vi "Array_filler.vi"() -> ()   [LabVIEW 2019]
panel:
  out "Indeks MAX":dbl[](array[numeric])
  out "Indeks MIN":dbl[](array[numeric])
  out "Rozmiar tablicy":dbl[](array[numeric])
  out "Suma":dbl
  out "Wartość MIN":dbl
  out "Wartość MAX":dbl
  in  "STOP":bool
  in  "Indeks kolumny":dbl
  in  "Indeks wiersza":dbl
  in  "Wypełnienie tablicy wstawianej":dbl
  out "Tablica wyjściowa":dbl[][](array[numeric])
  out "Tablica wstawiana":dbl[][](array[numeric])
  in  "Wprowadzanie danych":dbl[][](array[numeric])
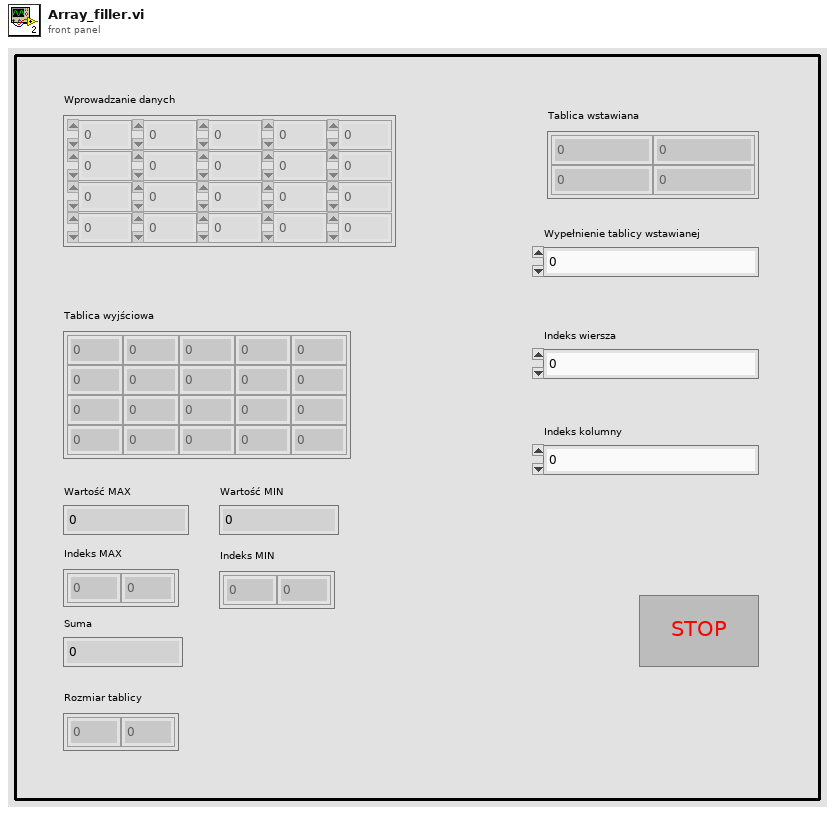
[diagram p1: front panel]
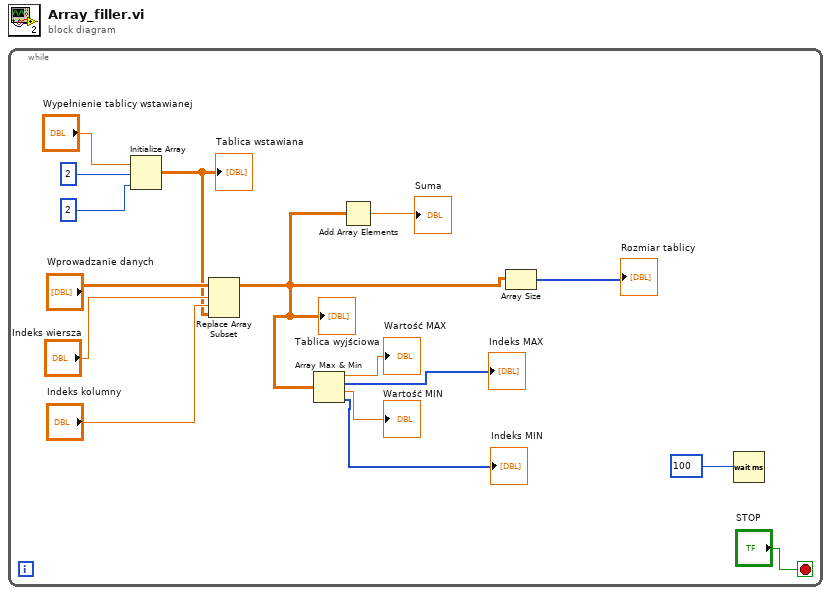
[diagram p0: block diagram]
diagram:
  n1 = while {
    stop <- "STOP" stop-if-true
    n2 = Initialize Array("Wypełnienie tablicy wstawianej", 2, 2) -> (w10:dbl[][])
    "Tablica wstawiana" <- w10
    n3 = Replace Array Subset(array="Wprowadzanie danych", new element=w10, index (row)="Indeks wiersza", index (col)="Indeks kolumny") -> (w6:dbl[][])
    "Tablica wyjściowa" <- w6
    n4 = Array Max & Min(array=w6) -> (max value=→"Wartość MAX":dbl, max index (indices)=→"Indeks MAX":i32[], min value=→"Wartość MIN":dbl, min index (indices)=→"Indeks MIN":i32[])
    n5 = Add Array Elements(numeric array=w6) -> (sum=→"Suma":dbl)
    n6 = Array Size(array=w6) -> (size(s)=→"Rozmiar tablicy":i32[])
    n7 = Wait (ms)(milliseconds to wait=100) -> ()  [unwired: 1 out]
  }
